vi "Untitled 1.vi"() -> ()   [LabVIEW 2023]
panel:
  in  "Numeric 7":i32
  out "appended array":dbl[][](array[numeric])
  out "Numeric 6":dbl
  in  "Array":dbl[][](array[numeric])
  out "Numeric 5":i32
  out "Numeric 4":i32
  out "Numeric 3":i32
  out "Numeric 2":i32
  out "Numeric":i32
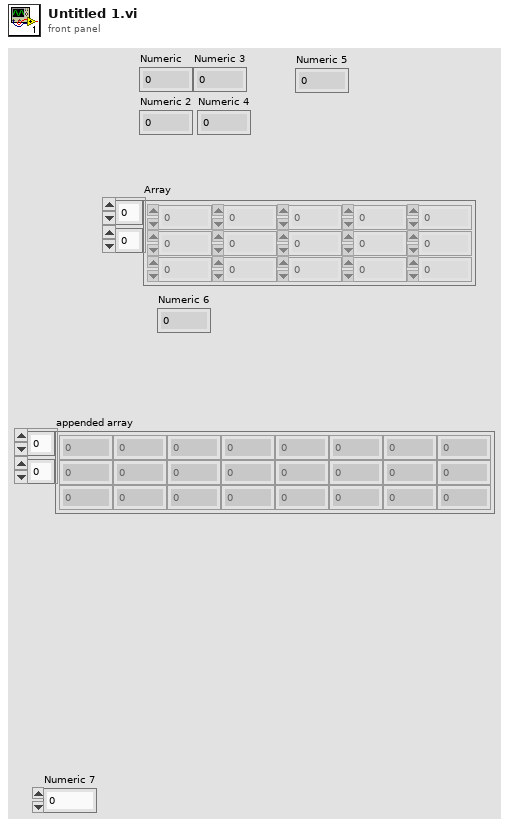
[diagram p1: front panel]
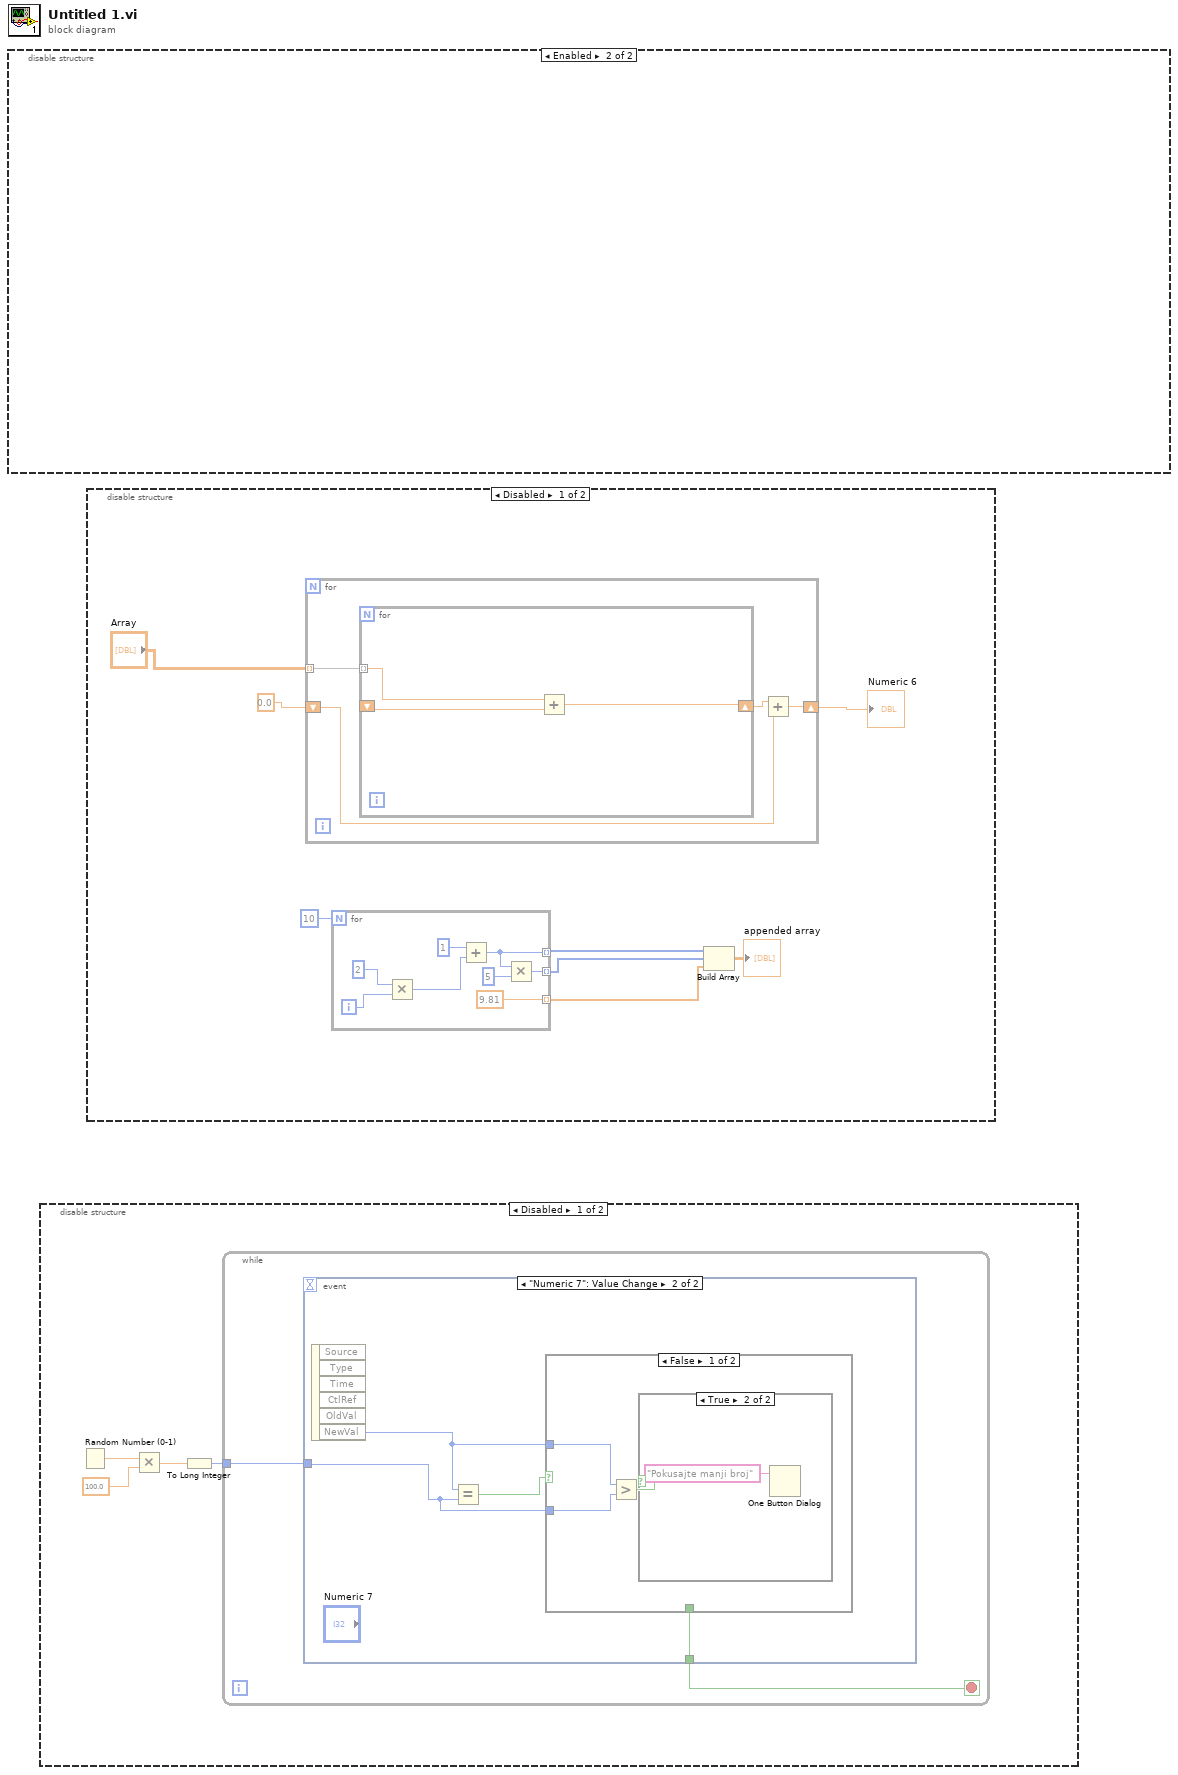
[diagram p0: block diagram]
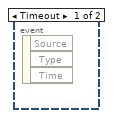
[diagram p2: hidden frame]
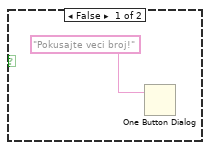
[diagram p3: hidden frame]
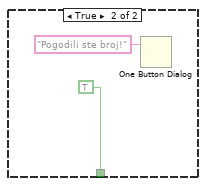
[diagram p4: hidden frame]
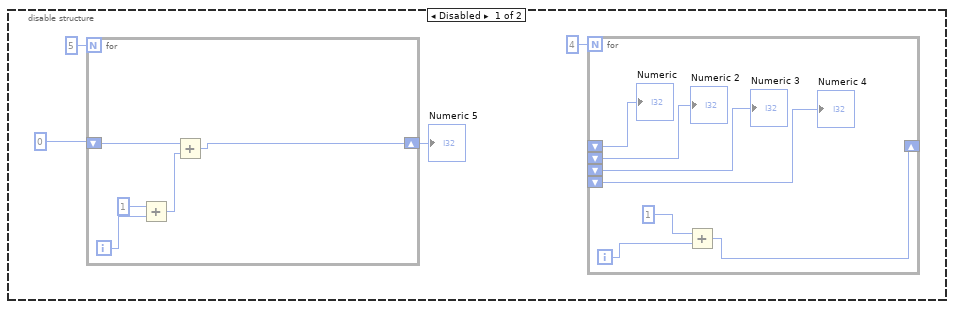
[diagram p7: hidden frame]
diagram:
  n1 = disable-structure shown="Enabled" {
    frame Disabled {
      n2 = for {
        N: 5 -> [_]
        shift-right: [w12] -> w1
        shift-left: 0 -> [w16]
        i -> [w15]
        n3 = Add(x=1, y=w15) -> (x+y=w13:i32)
        n4 = Add(x=w16, y=w13) -> (x+y=w12:i32)
      }
      "Numeric 5" <- w1
      n5 = for {
        N: 4 -> [_]
        shift-right: [w7] -> _
        shift-left: _ -> [w11]
        shift-left: _ -> [w10]
        shift-left: _ -> [w9]
        shift-left: _ -> [w8]
        i -> [w6]
        n6 = Add(x=1, y=w6) -> (x+y=w7:i32)
        "Numeric" <- w11
        "Numeric 2" <- w10
        "Numeric 3" <- w9
        "Numeric 4" <- w8
      }
    }
    frame Enabled {
    }
  }
  n7 = disable-structure shown="Disabled" {
    frame Disabled {
      n8 = Random Number (0-1)() -> (number: 0 to 1=w20:dbl)
      n9 = Multiply(x=w20, y=100.0) -> (x*y=w18:dbl)
      n10 = To Long Integer(number=w18) -> (32bit integer=w17:i32)
      n11 = while {
        tunnel: w17 -> [w22]
        stop <- w21 stop-if-true
        n12 = event shown="[1] \"Numeric 7\": Value Change" {
          selector: _ -> [_ _]
          dyn-events: _ -> [_ _]
          timeout: _ -> [_ _]
          tunnel: w22 -> [_ w23]
          tunnel: [_ w25] -> w21
          event Timeout {
            n13 = event-data() -> ()  [unwired: 1 in, 3 out]
          }
          event "Numeric 7": Value Change {
            n14 = event-data() -> ("NewVal"=w24:i32)  [unwired: 1 in, 5 out]
            n15 = Equal?(x=w24, y=w23) -> (x = y?=w26:bool)
            n16 = case shown="False" w26 {
              tunnel: [_ TRUE] -> w25
              tunnel: w24 -> [w28 _]
              tunnel: w23 -> [w27 _]
              frame False {
                n17 = Greater?(x=w28, y=w27) -> (0:w29:bool)
                n18 = case shown="True" w29 {
                  frame False {
                    n19 = One Button Dialog(message="Pokusajte veci broj!") -> ()  [unwired: 1 in, 1 out]
                  }
                  frame True {
                    n20 = One Button Dialog(message="Pokusajte manji broj") -> ()  [unwired: 1 in, 1 out]
                  }
                }
              }
              frame True {
                n21 = One Button Dialog(message="Pogodili ste broj!") -> ()  [unwired: 1 in, 1 out]
              }
            }
          }
        }
      }
    }
    frame Enabled {
    }
  }
  n22 = disable-structure shown="Disabled" {
    frame Disabled {
      n23 = for {
        shift-right: [w52] -> w39
        shift-left: 0.0 -> [w51]
        tunnel: "Array" -> [w53] mode=indexing
        n24 = for {
          shift-right: [w56] -> w50
          shift-left: _ -> [w55]
          tunnel: w53 -> [w54] mode=indexing
          n25 = Add(x=w54, y=w55) -> (x+y=w56:dbl)
        }
        n26 = Add(x=w50, y=w51) -> (x+y=w52:dbl)
      }
      "Numeric 6" <- w39
      n27 = for {
        N: 10 -> [_]
        tunnel: [w44] -> w35 mode=indexing
        tunnel: [9.81] -> w36 mode=indexing
        tunnel: [w42] -> w38 mode=indexing
        i -> [w49]
        n28 = Multiply(x=2, y=w49) -> (x*y=w47:i32)
        n29 = Add(x=1, y=w47) -> (x+y=w44:i32)
        n30 = Multiply(x=w44, y=5) -> (x*y=w42:i32)
      }
      n31 = Build Array(w35, w38, w36) -> (→"appended array":dbl[][])
    }
    frame Enabled {
    }
  }
